vi "LogDirFileName Value Change.vi"(4 "Linux Log Directory":string caption="Log Directory", 6 "Windows Log Directory":path, 7 "Control Refs":T1, 8 "File Name":string, 9 "Linux Paths?":bool, 10 "Event References":T2, 11 "References":T9) -> (0 "error out":errorcluster, 2 "Logging File Path":string)   [LabVIEW 2015, in "TDMS datalogger editor node.lvclass"]
uses:
  TDMS datalogger editor node.lvclass
  <vilib>/NI/DCAF/Tag Editor Core/Table API/Table Manager/object ref.ctl
  <vilib>/NI/DCAF/Tag Editor Core/Configuration Editor/Classes/Engine Parent/Engine Parent Editor Node.lvclass
  <vilib>/NI/DCAF/Tag Editor Core/Configuration Editor/Classes/Module editor node/module editor node.lvclass
  <vilib>/NI/DCAF/Tag Editor Core/Table API/Table Manager/references.ctl
  <vilib>/NI/Configuration Framework/Node/StopEvent.ctl
  <vilib>/NI/Configuration Framework/Node/RefreshUIEvent.ctl
  <vilib>/NI/Configuration Framework/Node/CacheState.ctl
  <vilib>/NI/Configuration Framework/Node/NodeChangeEvent.ctl
  <vilib>/NI/Configuration Framework/Node/NodeRef.ctl
  <vilib>/NI/Configuration Framework/Node/NISE_CEF_Node.lvclass
  <vilib>/NI/DCAF/Tag Editor Core/Table API/Available Tag Menu/channel action event.ctl
  <vilib>/NI/DCAF/Tag Editor Core/Table API/Available Tag Menu/dialog output action.ctl
  <vilib>/NI/Tag Bus Module Framework/channel/TBM channel.lvclass
  <vilib>/NI/Tag Bus/tag/tag descriptor.lvclass
  <vilib>/NI/DCAF/Tag Editor Core/Table API/Table Manager/Call Back Ref Type Def.ctl
  <vilib>/NI/AMC/Message Queue.ctl
  <vilib>/NI/AMC/Message.ctl
  <vilib>/NI/Tools/Keyed Array/KeyedArray.ctl
  <vilib>/NI/Configuration Framework/Node/UserEventRef.ctl
  <vilib>/NI/Configuration Framework/Controls/EventCluster.ctl
  Control Refs.ctl
  TDMS datalogger editor node.lvclass/TDMS datalogger editor node.ctl
  module/configuration/TDMS datalogger configuration.lvclass/TDMS datalogger configuration.ctl
  module/configuration/Write log name.vi
  module/configuration/Write log directory.vi
  module/configuration/Write log file path.vi
  <vilib>/regexp/Match Regular Expression.xnode
  module/configuration/TDMS datalogger configuration.lvclass
  <vilib>/NI/DCAF/Tag Editor Core/Table API/Table Manager/Table Manager.lvclass
  <vilib>/NI/DCAF/Tag Editor Core/Table API/Table Manager.lvlib
  <vilib>/NI/Tools/Keyed Array/Tools_KeyedArray.lvlib
  <vilib>/NI/AMC/AMC.lvlib
  <vilib>/NI/Configuration Framework/NISE_CEF_TreeControl.lvlib
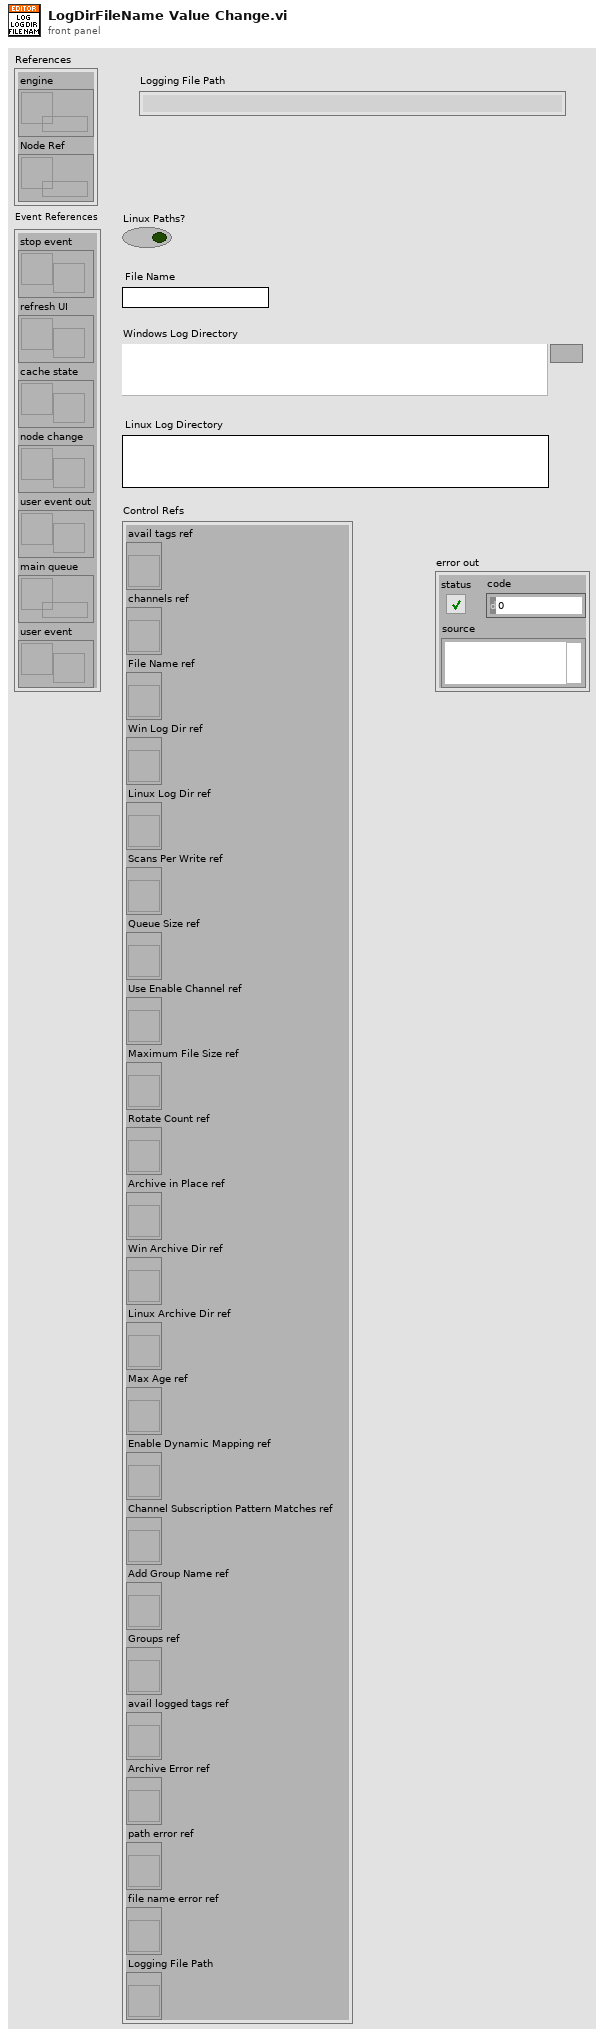
[diagram p1: front panel]
types:
  T1 = typedef "Control Refs.ctl" = cluster{"avail tags ref":refnum<vi>, "channels ref":refnum<vi>, "File Name ref":refnum<vi>, "Win Log Dir ref":refnum<vi>, "Linux Log Dir ref":refnum<vi>, "Scans Per Write ref":refnum<vi>, "Queue Size ref":refnum<vi>, "Use Enable Channel ref":refnum<vi>, "Maximum File Size ref":refnum<vi>, "Rotate Count ref":refnum<vi>, "Archive in Place ref":refnum<vi>, "Win Archive Dir ref":refnum<vi>, "Linux Archive Dir ref":refnum<vi>, "Max Age ref":refnum<vi>, "Enable Dynamic Mapping ref":refnum<vi>, "Channel Subscription Pattern Matches ref":refnum<vi>, "Add Group Name ref":refnum<vi>, "Groups ref":refnum<vi>, "avail logged tags ref":refnum<vi>, "Archive Error ref":refnum<vi>, "path error ref":refnum<vi>, "file name error ref":refnum<vi>, "Logging File Path":refnum<vi>}
  T2 = typedef "Table Manager.lvlib/Table Manager.lvclass/references.ctl" = cluster{"stop event":T3, "refresh UI":T4, "cache state":T5, "node change":T6, "user event out":refnum<user-event>, "main queue":T7, "user event":T8}
  T3 = typedef "NISE_CEF_Node.lvclass/StopEvent.ctl" = refnum<user-event>
  T4 = typedef "NISE_CEF_Node.lvclass/RefreshUIEvent.ctl" = refnum<user-event>
  T5 = typedef "NISE_CEF_Node.lvclass/CacheState.ctl" = refnum<user-event>
  T6 = typedef "NISE_CEF_Node.lvclass/NodeChangeEvent.ctl" = refnum<user-event>
  T7 = typedef "AMC.lvlib/Message Queue.ctl" = refnum<queue>
  T8 = typedef "NISE_CEF_Node.lvclass/UserEventRef.ctl" = refnum<user-event>
  T9 = typedef "Table Manager.lvlib/Table Manager.lvclass/object ref.ctl" = cluster{"engine":refnum<data-value>, "Node Ref":refnum<data-value>}
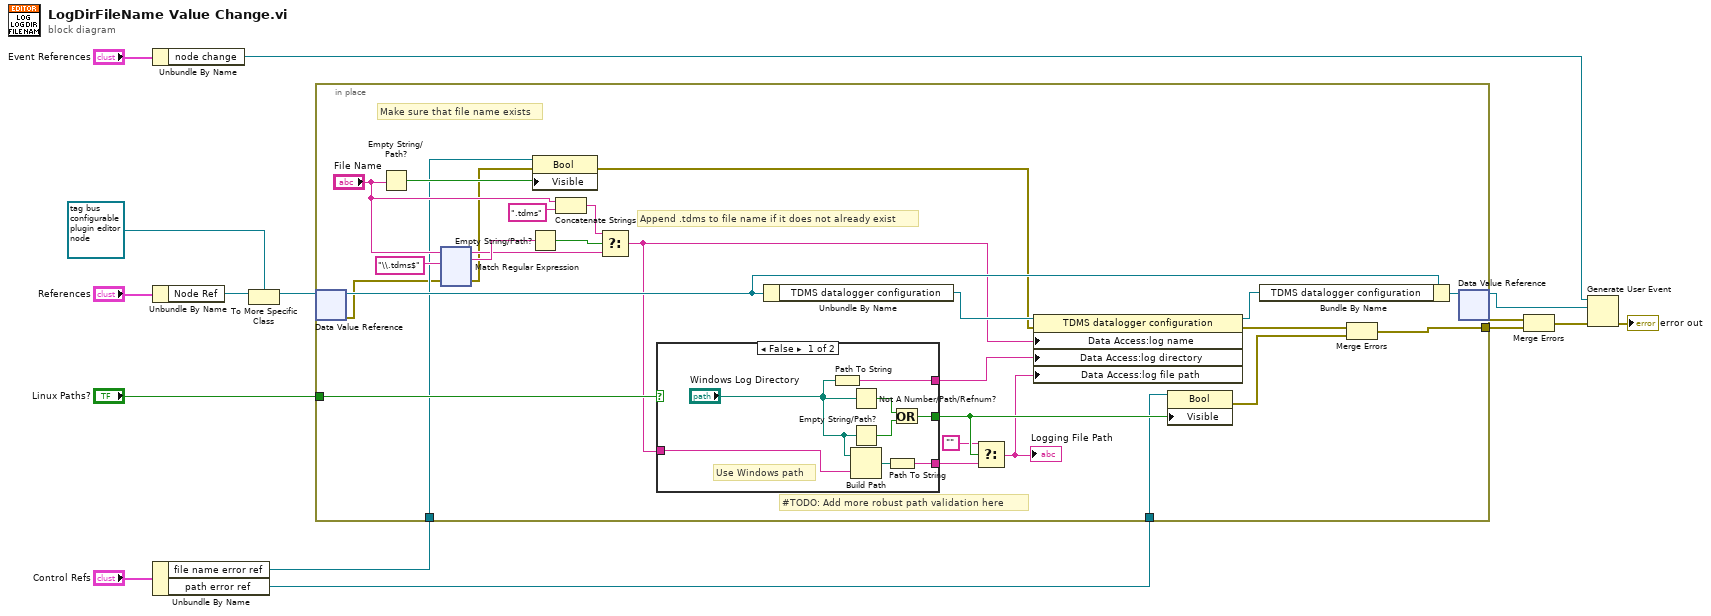
[diagram p0: block diagram]
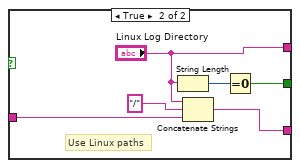
[diagram p2: hidden frame]
diagram:
  n1 = Unbundle By Name("Event References") -> ("node change"=w10:T6)
  n2 = Unbundle By Name("References") -> ("Node Ref"=w13:refnum<data-value>)
  n3 = Unbundle By Name("Control Refs") -> ("file name error ref"=w1:refnum<vi>, "path error ref"=w2:refnum<vi>)
  n4 = To More Specific Class(target class=refnum<data-value> refnum ("data value reference"), reference=w13) -> (specific class reference=w11:refnum<data-value>)  [unwired: 1 in, 1 out]
  n5 = in-place {
    in-place-border: [w22] -> w9
    in-place-border: "Linux Paths?" -> [w36]
    in-place-border: w2 -> [w23]
    in-place-border: w1 -> [w21]
    # "Append .tdms to file name if it does not already exist"
    # "Make sure that file name exists"
    # "#TODO: Add more robust path validation here"
    n6 = in-place-dvr #1(w11) -> (w37:refnum<class "TDMS datalogger editor node.lvclass">, w19:errorcluster)
    n7 = Empty String/Path?(string/path="File Name") -> (empty?=w32:bool)
    n8 = xnode "Match Regular Expression"("input string"="File Name", "regular expression"="\\.tdms$", "error in"=w19) -> ("whole match"=w34:string, "error out"=w18:errorcluster)  [unwired: 3 in, 3 out]
    n9 = Empty String/Path?(string/path=w34) -> (empty?=w33:bool)
    n10 = property on="Property Node" class="Bool"(reference=w21, error in=w18, "Visible"=w32) -> (error out=w17:errorcluster)  [unwired: 1 out]
    n11 = Concatenate Strings("File Name", ".tdms" ("string")) -> (w30:string)
    n12 = Select(t=w30, s=w33, f="File Name") -> (s? t:f=w25:string)
    n13 = case shown="False" w36 {
      tunnel: [w161 w168] -> w28
      tunnel: [w160 "Linux Log Directory"] -> w24
      tunnel: w25 -> [w158 w166]
      tunnel: [w156 w164] -> w27
      frame False {
        # "Use Windows path"
        n14 = Path To String(path="Windows Log Directory") -> (string=w160:string)
        n15 = Not A Number/Path/Refnum?(number/path/refnum="Windows Log Directory") -> (NaN/Path/Refnum?=w162:bool)
        n16 = Empty String/Path?(string/path="Windows Log Directory") -> (empty?=w163:bool)
        n17 = Build Path(base path="Windows Log Directory", name or relative path=w158) -> (appended path=w157:path)
        n18 = Path To String(path=w157) -> (string=w156:string)
        n19 = Or(x=w162, y=w163) -> (x .or. y?=w161:bool)
      }
      frame True {
        # "Use Linux paths"
        n20 = String Length(string="Linux Log Directory") -> (length=w169:i32)
        n21 = Concatenate Strings("Linux Log Directory", "/" ("string"), w166) -> (w164:string)
        n22 = Equal To 0?(x=w169) -> (x = 0?=w168:bool)
      }
    }
    n23 = Unbundle By Name(w37) -> ("TDMS datalogger configuration"=w40:refnum<class "TDMS datalogger configuration.lvclass">)
    n24 = Select(t="", s=w28, f=w27) -> (s? t:f=w16:string)
    "Logging File Path" <- w16
    n25 = property class="TDMS datalogger configuration"(reference=w40, error in=w17, "Data Access:log name"=w25, "Data Access:log directory"=w24, "Data Access:log file path"=w16) -> (reference out=w39:refnum<class "TDMS datalogger configuration.lvclass">, error out=w41:errorcluster)
    n26 = property on="Property Node" class="Bool"(reference=w23, "Visible"=w28) -> (error out=w20:errorcluster)  [unwired: 1 in, 1 out]
    n27 = Bundle By Name(cluster=w37, "TDMS datalogger configuration"=w39) -> (w38:refnum<class "TDMS datalogger editor node.lvclass">)
    n28 = Merge Errors(w41, w20) -> (w22:errorcluster)
    n29 = in-place-dvr #1(w38) -> (w15:refnum<data-value>, w7:errorcluster)
  }
  n30 = Merge Errors(w7, w9) -> (w8:errorcluster)
  n31 = Generate User Event(user event=w10, event data cluster=w15, error in=w8) -> (error out=→"error out":errorcluster)  [unwired: 1 in, 1 out]
